vi "Create Template.vi"(8 "error in (no error)":errorcluster, 11 "eLab in":refnum<class "PL eLabFTW Client.lvclass">) -> (0 "error out":errorcluster, 2 "template id":u32, 3 "eLab out":refnum<class "PL eLabFTW Client.lvclass">)   [LabVIEW 2015, in "PL eLabFTW Client.lvclass"]
doc: "Creates new template and returns new template id."
uses:
  PL eLabFTW Client.lvclass
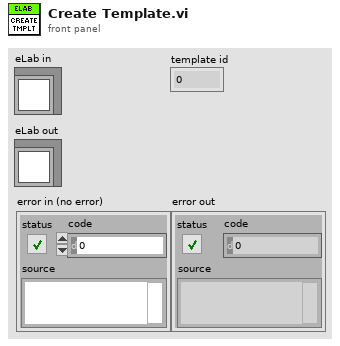
[diagram p1: front panel]
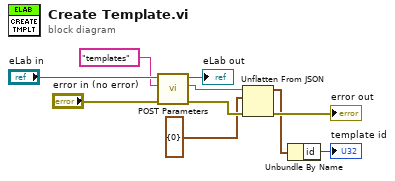
[diagram p0: block diagram]
diagram:
  n1 = call "POST Parameters.vi"("error in (no error)"="error in (no error)", "relative URL"="templates" ("format string"), "eLab in"="eLab in") -> ("error out"=w7:errorcluster, "response body"=w3:string, "eLab out"=→"eLab out":refnum<class "PL eLabFTW Client.lvclass">)  [unwired: 6 in]
  n2 = Unflatten From JSON(JSON string=w3, type and defaults=cluster{"id":u32} {"id"=0}, error in (no error)=w7) -> (value=w4:cluster{"id":u32}, error out=→"error out":errorcluster)  [unwired: 4 in]
  n3 = Unbundle By Name(w4) -> ("id"=→"template id":u32)
